vi "nPoints Path.vi"(8 "error in (no error)":errorcluster, 11 "name or relative path":string) -> (0 "error out":errorcluster, 3 "File path":path)   [LabVIEW 2013]
panel:
  in  "Use Dialog (F)":bool
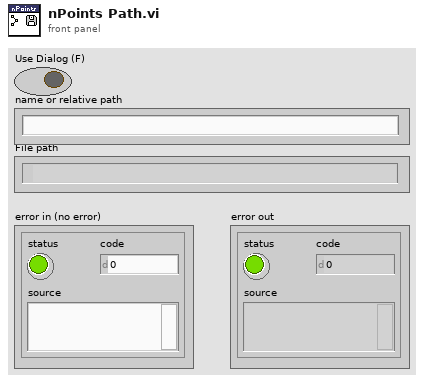
[diagram p1: front panel]
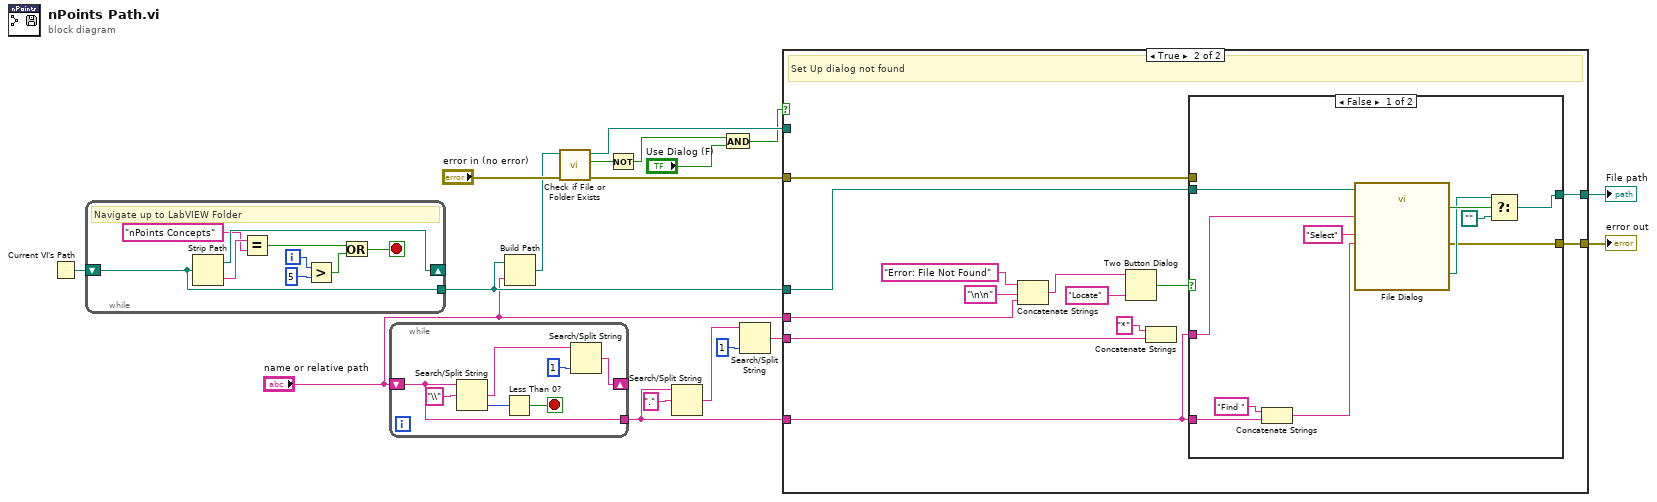
[diagram p0: block diagram]
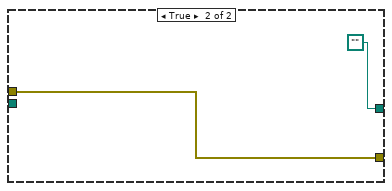
[diagram p3: hidden frame]
diagram:
  n1 = Current VI's Path() -> (path=w16:path)
  n2 = while {
    shift-right: [w27] -> _
    shift-left: w16 -> [w24]
    tunnel: [w24] -> w8
    i -> [w22]
    stop <- w19 stop-if-true
    # "Navigate up to LabVIEW Folder"
    n3 = Strip Path(path=w24) -> (stripped path=w27:path, name=w26:string)
    n4 = Equal?(x=w26, y="nPoints Concepts" ("name or relative path")) -> (x = y?=w23:bool)
    n5 = Greater?(x=w22, y=5) -> (0:w20:bool)
    n6 = Or(x=w23, y=w20) -> (x .or. y?=w19:bool)
  }
  n7 = while {
    shift-right: [w29] -> _
    shift-left: "name or relative path" -> [w28]
    tunnel: [w28] -> w4
    stop <- w32 stop-if-true
    n8 = Search/Split String(string=w28, search string/char (-)="\\") -> (match + rest of string=w31:string, offset of match=w33:i32)  [unwired: 1 in, 1 out]
    n9 = Less Than 0?(x=w33) -> (x < 0?=w32:bool)
    n10 = Search/Split String(string=w31, offset (0)=1) -> (match + rest of string=w29:string)  [unwired: 1 in, 2 out]
  }
  n11 = Build Path(base path=w8, name or relative path="name or relative path") -> (appended path=w12:path)
  n12 = call <vilib>:"Check if File or Folder Exists.vi"("error in (no error)"="error in (no error)", "path"=w12) -> ("error out"=w14:errorcluster, "file or folder exists?"=w15:bool, "dup path"=w13:path)  [unwired: 7 in]
  n13 = Not(x=w15) -> (.not. x?=w6:bool)
  n14 = Search/Split String(string=w4, search string/char (-)=".") -> (match + rest of string=w3:string)  [unwired: 1 in, 2 out]
  n15 = And(x=w6, y="Use Dialog (F)") -> (x .and. y?=w10:bool)
  n16 = Search/Split String(string=w3, offset (0)=1) -> (match + rest of string=w1:string)  [unwired: 1 in, 2 out]
  n17 = case shown="True" w10 {
    tunnel: [w35 w39] -> w11
    tunnel: w13 -> [w36 _]
    tunnel: w14 -> [w35 w38]
    tunnel: "name or relative path" -> [_ w49]
    tunnel: [w36 w42] -> w18
    tunnel: w8 -> [_ w43]
    tunnel: w4 -> [_ w37]
    tunnel: w1 -> [_ w41]
    frame False {
      # "Open set up dialog, and bring to front"
    }
    frame True {
      # "Set Up dialog not found"
      n18 = Concatenate Strings("Error: File Not Found" ("message"), "\n\n" ("string"), w49) -> (w46:string)
      n19 = Two Button Dialog(message=w46, 1:"Locate" ("F button name (\"Cancel\")")) -> (T button?=w44:bool)  [unwired: 1 in]
      n20 = Concatenate Strings("*" ("string"), w41) -> ()  [unwired: 1 out]
      n21 = case shown="False" w44 {
        tunnel: w43 -> [w60 _]
        tunnel: [w58 path ""] -> w42
        tunnel: w37 -> [w53 _]
        tunnel: w37 -> [w52 _]
        tunnel: [w50 w61] -> w39
        tunnel: w38 -> [_ w61]
        frame False {
          n22 = Concatenate Strings("Find " ("prompt"), w53) -> (w51:string)
          n23 = call "File Dialog"("start path"=w60, "prompt"=w51, "button label"="Select", "pattern (all files)"=w52) -> ("selected path"=w56:path, "exists"=w57:bool, "error out"=w50:errorcluster)  [unwired: 8 in, 1 out]
          n24 = Select(t=w56, s=w57, f=path "") -> (s? t:f=w58:path)
        }
        frame True {
        }
      }
    }
  }
  "File path" <- w18
  "error out" <- w11
